vi "xijk_set_example.vi"(8 "error in":errorcluster, 9 "examples in":u8, 11 "Table of settings in":path[](array[path])) -> (0 "error out":errorcluster, 1 "project name":string, 5 "filepaths out":T2, 7 "spectra parameters out":T1={"Booleans"={"Notch filtering"=FALSE, "Unknown detector"=FALSE, "Dual band filters"=FALSE, "Dual emission by cubes"=FALSE, "FRET"=FALSE}, "Integers"={"Light source"=0, "Number of fluorophores"=0, "Wavelength of laser (nm) 1"=0, "Broadness of laser (nm) 1"=0, "Wavelength of laser (nm) 2"=0, "Broadness of laser (nm) 2"=0, "Template"=1}, "Doubles"={"Molar extinction 1"=1.0, "Molar extinction 2"=1.0, "Quantum efficiency 1"=1.0, "Quantum efficiency 2"=1.0}})   [LabVIEW 2010]
uses:
  Type Def/spectra_parameters.ctl
  Type Def/filepath.ctl
  <vilib>/Utility/file.llb/Read From Spreadsheet File (string).vi
panel:
  in  "spectra parameters":T1={"Booleans"={"Notch filtering"=FALSE, "Unknown detector"=FALSE, "Dual band filters"=FALSE, "Dual emission by cubes"=FALSE, "FRET"=FALSE}, "Integers"={"Light source"=0, "Number of fluorophores"=0, "Wavelength of laser (nm) 1"=0, "Broadness of laser (nm) 1"=0, "Wavelength of laser (nm) 2"=0, "Broadness of laser (nm) 2"=0, "Template"=1}, "Doubles"={"Molar extinction 1"=1.0, "Molar extinction 2"=1.0, "Quantum efficiency 1"=1.0, "Quantum efficiency 2"=1.0}}
  in  "filepaths":T2
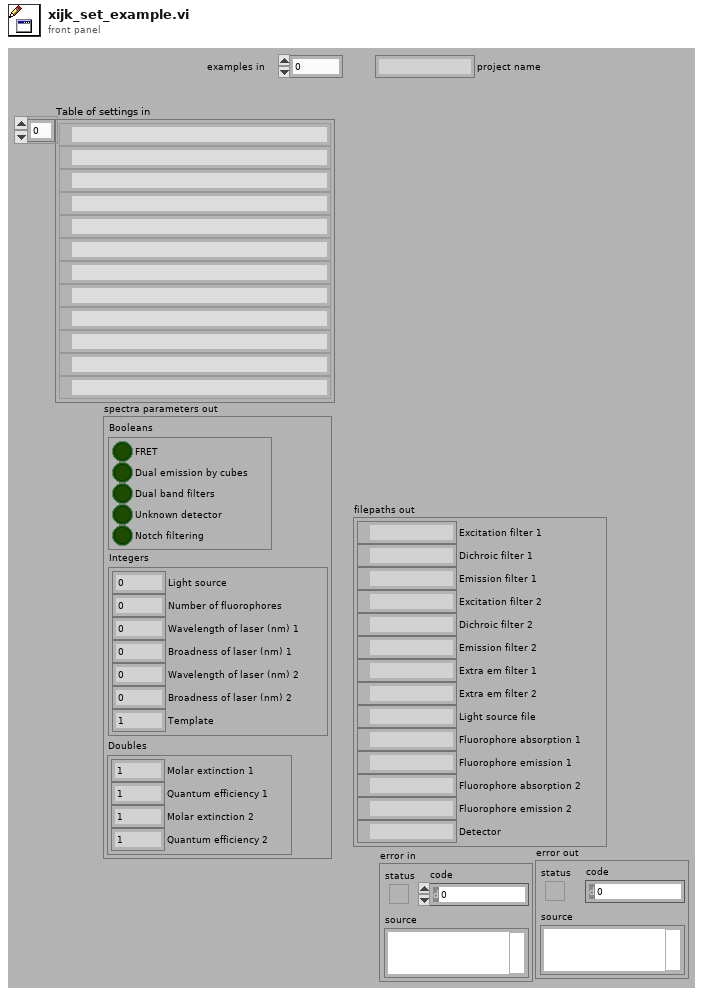
[diagram p1: front panel]
types:
  T1 = typedef "spectra_parameters.ctl" = cluster{"Booleans":cluster{"Notch filtering":bool, "Unknown detector":bool, "Dual band filters":bool, "Dual emission by cubes":bool, "FRET":bool}, "Integers":cluster{"Light source":u16, "Number of fluorophores":u16, "Wavelength of laser (nm) 1":u16, "Broadness of laser (nm) 1":u16, "Wavelength of laser (nm) 2":u16, "Broadness of laser (nm) 2":u16, "Template":u16}, "Doubles":cluster{"Molar extinction 1":dbl, "Molar extinction 2":dbl, "Quantum efficiency 1":dbl, "Quantum efficiency 2":dbl}}
  T2 = typedef "filepath.ctl" = cluster{"Excitation filter 1":path, "Dichroic filter 1":path, "Emission filter 1":path, "Excitation filter 2":path, "Dichroic filter 2":path, "Emission filter 2":path, "Extra em filter 1":path, "Extra em filter 2":path, "Light source file":path, "Fluorophore absorption 1":path, "Fluorophore emission 1":path, "Fluorophore absorption 2":path, "Fluorophore emission 2":path, "Detector":path}
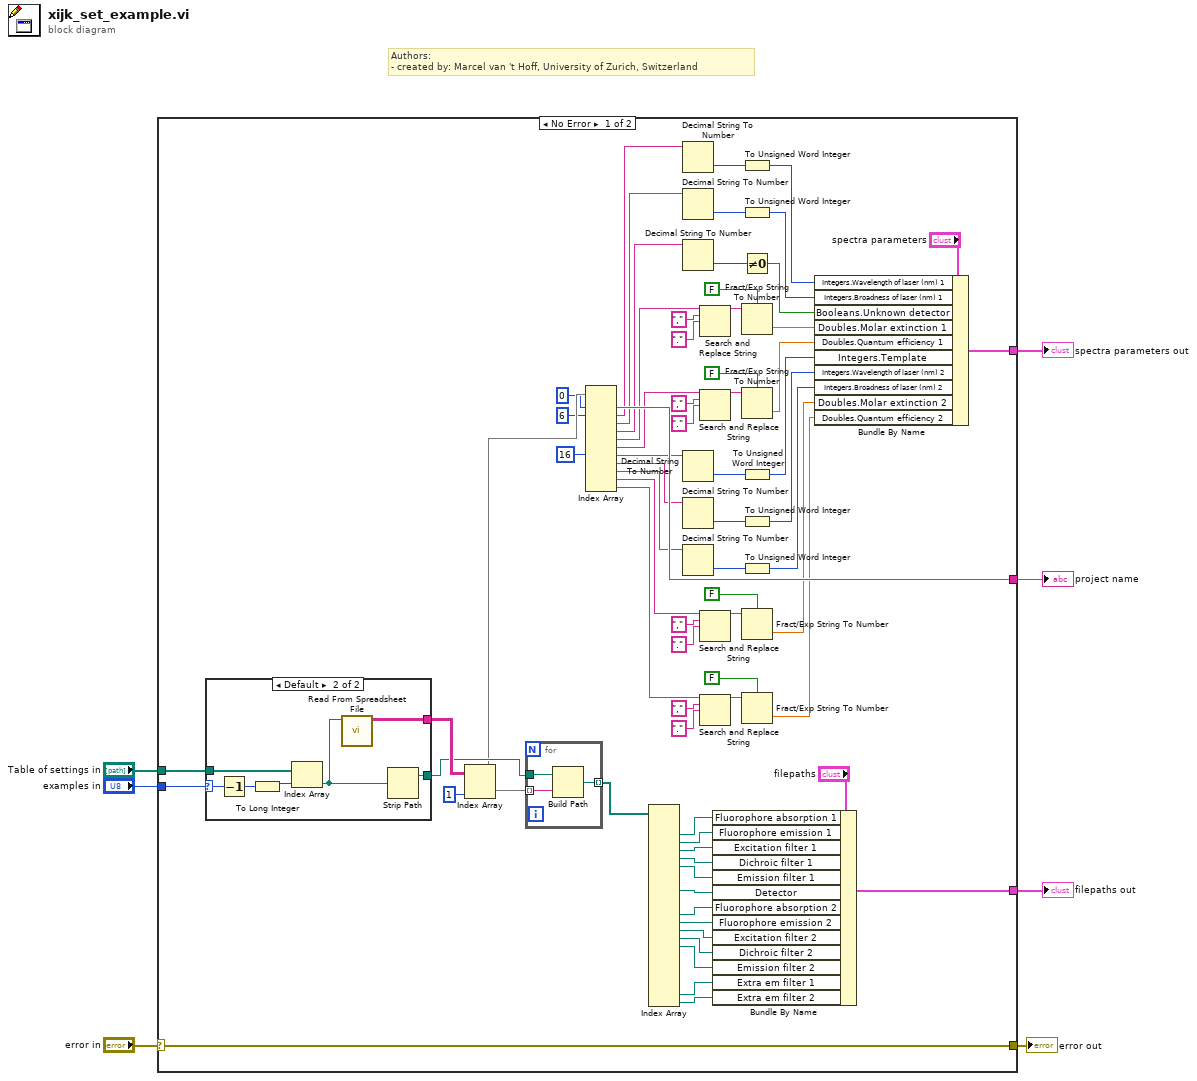
[diagram p0: block diagram]
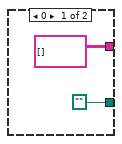
[diagram p2: hidden frame]
diagram:
  # "Authors: \n- created by: Marcel van 't Hoff, University of Zurich, Switzerland"
  n1 = case shown="No Error" "error in" {
    selector: "error in" -> [w8 w91]
    tunnel: "Table of settings in" -> [w78 _]
    tunnel: "examples in" -> [w77 _]
    tunnel: [w74 _] -> w5
    tunnel: [w68 _] -> w4
    tunnel: [w64 _] -> w3
    tunnel: [w8 w91] -> w1
    frame No Error {
      n2 = case shown="Default" w77 {
        selector: w77 -> [_ w86]
        tunnel: [string[][] [] ("all rows") w88] -> w76
        tunnel: [path "" w90] -> w72
        tunnel: w78 -> [_ w87]
        frame 0 {
        }
        frame Default {
          n3 = Decrement(x=w86) -> (x-1=w85:u8)
          n4 = To Long Integer(number=w85) -> (32bit integer=w84:i32)
          n5 = Index Array(array=w87, index=w84) -> (element=w89:path)
          n6 = call-poly <vilib>:"Read From Spreadsheet File.vi"("file path (dialog if empty)"=w89) -> ("all rows"=w88:string[][])  [unwired: 3 in, 7 out]
          n7 = Strip Path(path=w89) -> (stripped path=w90:path)  [unwired: 1 out]
        }
      }
      n8 = Index Array(array=w76, index (col)=1 ("disabled index (col)")) -> (element=w70:string[])  [unwired: 1 in]
      n9 = for {
        tunnel: w70 -> [w81] mode=indexing
        tunnel: w72 -> [w80]
        tunnel: [w79] -> w71 mode=indexing
        n10 = Build Path(base path=w80, name or relative path=w81) -> (appended path=w79:path)
      }
      n11 = Index Array(array=w70, index #1=0 ("index"), index #2=6 ("index"), index #7=16 ("index")) -> (element #1=w68:string, element #2=w66:string, element #3=w62:string, element #4=w60:string, element #5=w55:string, element #6=w43:string, element #7=w42:string, element #8=w41:string, element #9=w40:string, element #10=w34:string, element #11=w30:string)  [unwired: 8 in]
      n12 = Index Array(array=w71) -> (element #2=w13:path, element #3=w14:path, element #4=w15:path, element #5=w16:path, element #6=w17:path, element #9=w18:path, element #12=w19:path, element #13=w20:path, element #14=w21:path, element #15=w22:path, element #16=w23:path, element #22=w24:path, element #23=w25:path)  [unwired: 23 in, 10 out]
      n13 = Decimal String To Number(string=w66) -> (number=w63:i32)  [unwired: 3 out]
      n14 = Decimal String To Number(string=w62) -> (number=w61:i32)  [unwired: 3 out]
      n15 = Decimal String To Number(string=w60) -> (number=w59:i32)  [unwired: 3 out]
      n16 = Decimal String To Number(string=w42) -> (number=w52:i32)  [unwired: 3 out]
      n17 = Decimal String To Number(string=w41) -> (number=w50:i32)  [unwired: 3 out]
      n18 = Decimal String To Number(string=w40) -> (number=w49:i32)  [unwired: 3 out]
      n19 = Search and Replace String(input string=w55, search string="," ("chaîne recherchée"), replace string="." ("chaîne de remplacement (\"\")")) -> (result string=w54:string)  [unwired: 1 in, 7 out]
      n20 = Search and Replace String(input string=w43, search string="," ("chaîne recherchée"), replace string="." ("chaîne de remplacement (\"\")")) -> (result string=w48:string)  [unwired: 1 in, 7 out]
      n21 = Search and Replace String(input string=w34, search string="," ("chaîne recherchée"), replace string="." ("chaîne de remplacement (\"\")")) -> (result string=w33:string)  [unwired: 1 in, 7 out]
      n22 = Search and Replace String(input string=w30, search string="," ("chaîne recherchée"), replace string="." ("chaîne de remplacement (\"\")")) -> (result string=w37:string)  [unwired: 1 in, 7 out]
      n23 = Bundle By Name(cluster="filepaths", "Fluorophore absorption 1"=w13, "Fluorophore emission 1"=w14, "Excitation filter 1"=w15, "Dichroic filter 1"=w16, "Emission filter 1"=w17, "Detector"=w18, "Fluorophore absorption 2"=w19, "Fluorophore emission 2"=w20, "Excitation filter 2"=w21, "Dichroic filter 2"=w22, "Emission filter 2"=w23, "Extra em filter 1"=w24, "Extra em filter 2"=w25) -> (w74:T2)
      n24 = To Unsigned Word Integer(number=w63) -> (unsigned 16bit integer=w10:u16)
      n25 = To Unsigned Word Integer(number=w61) -> (unsigned 16bit integer=w9:u16)
      n26 = Not Equal To 0?(x=w59) -> (x != 0?=w58:bool)
      n27 = Fract/Exp String To Number(use system decimal point (T)=FALSE ("utiliser le séparateur décimal du système (V)"), string=w54) -> (number=w53:dbl)  [unwired: 3 out]
      n28 = Fract/Exp String To Number(use system decimal point (T)=FALSE ("utiliser le séparateur décimal du système (V)"), string=w48) -> (number=w45:dbl)  [unwired: 3 out]
      n29 = To Unsigned Word Integer(number=w52) -> (unsigned 16bit integer=w51:u16)
      n30 = To Unsigned Word Integer(number=w50) -> (unsigned 16bit integer=w12:u16)
      n31 = To Unsigned Word Integer(number=w49) -> (unsigned 16bit integer=w11:u16)
      n32 = Fract/Exp String To Number(use system decimal point (T)=FALSE ("utiliser le séparateur décimal du système (V)"), string=w33) -> (number=w32:dbl)  [unwired: 3 out]
      n33 = Fract/Exp String To Number(use system decimal point (T)=FALSE ("utiliser le séparateur décimal du système (V)"), string=w37) -> (number=w31:dbl)  [unwired: 3 out]
      n34 = Bundle By Name(cluster="spectra parameters", "Integers.Wavelength of laser (nm) 1"=w10, "Integers.Broadness of laser (nm) 1"=w9, "Booleans.Unknown detector"=w58, "Doubles.Molar extinction 1"=w53, "Doubles.Quantum efficiency 1"=w45, "Integers.Template"=w51, "Integers.Wavelength of laser (nm) 2"=w12, "Integers.Broadness of laser (nm) 2"=w11, "Doubles.Molar extinction 2"=w32, "Doubles.Quantum efficiency 2"=w31) -> (w64:T1)
    }
    frame Error {
    }
  }
  "project name" <- w4
  "spectra parameters out" <- w3
  "filepaths out" <- w5
  "error out" <- w1
